vi "Unbundle Command.vi"(8 "error in (no error)":errorcluster, 10 "command":T3={"Command"=enum."Receive", "Command Parameters"={"arg1"=0, "arg2"=0}}, 11 "Transceiver Thread in":refnum<class "Transceiver Thread.lvclass">) -> (0 "error out":errorcluster, 1 "command":T1=enum."Receive", 2 "command parameters":T2, 3 "Transceiver Thread out":refnum<class "Transceiver Thread.lvclass">)   [LabVIEW 2017, in "Data Sharing Framework Core.lvlib" / "Data Sharing Framework Engine.lvlib" / "Transceiver Thread.lvclass"]
uses:
  Transceiver Thread.lvclass
  Interfaces/Transceiver Interface/Command Data.ctl
  Interfaces/Transceiver Interface/Command.ctl
  Interfaces/Transceiver Interface/Command Parameters.ctl
  Interfaces/Transceiver Interface/Transceiver Interface.lvclass
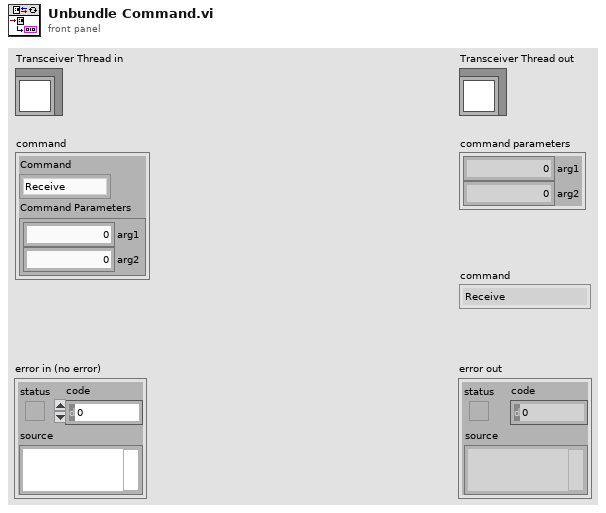
[diagram p1: front panel]
types:
  T1 = typedef "Data Sharing Framework Core.lvlib/Data Sharing Framework Engine.lvlib/Transceiver Interface.lvclass/Command.ctl" = enum8{"Set Base Pointer", "Receive", "Transmit", "Shutdown"}
  T2 = typedef "Data Sharing Framework Core.lvlib/Data Sharing Framework Engine.lvlib/Transceiver Interface.lvclass/Command Parameters.ctl" = cluster{"arg1":u64, "arg2":u64}
  T3 = typedef "Data Sharing Framework Core.lvlib/Data Sharing Framework Engine.lvlib/Transceiver Interface.lvclass/Command Data.ctl" = cluster{"Command":T1, "Command Parameters":T2}
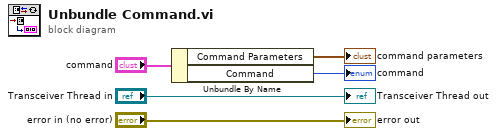
[diagram p0: block diagram]
diagram:
  n1 = Unbundle By Name("command") -> ("Command Parameters"=→"command parameters":T2, "Command"=→"command":T1)
  "error out" <- "error in (no error)"
  "Transceiver Thread out" <- "Transceiver Thread in"
